vi "MAT_Footer.vi"(6 "byte order":T2(ring)=enum."little-endian", 9 "# plots":i32=6, 10 "frequency":dbl=40000.0, 11 "npts":i32=32768) -> (3 "String":string)   [LabVIEW 2022 SP3]
uses:
  miDataType.ctl
panel:
  out "Array":T1(array[cluster])
  out "WoodhouseCheck":bool
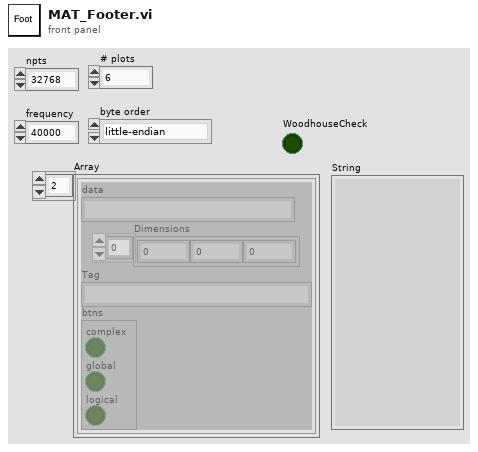
[diagram p1: front panel]
types:
  T1 = cluster{"data":string, "Dimensions":i32[], "Tag":string, "btns":cluster{"complex":bool, "global":bool, "logical":bool}}[]
  T2 = enum16{"big-endian, network order", "native, host order", "little-endian"}
  T3 = cluster{"name":string, "Dimensions":i32[], "Tag":string, "btns":cluster{"complex":bool, "global":bool, "logical":bool}}[]
  T4 = typedef "miDataType.ctl" = enum16{"illegal", "miINT8", "miUINT8", "miINT16", "miUINT16", "miINT32", "miUINT32", "miSINGLE", "--", "miDOUBLE", "---", "----", "miINT64", "miUINT64", "miMATRIX", "miCOMPRESSED", "miUTF8", "miUTF16", "miUTF32", "udefined"}
  T5 = cluster{"data":string, "Dimensions":i32[], "Tag":cluster{"Data Type":T4, "# bytes":u32, "data":string}, "btns":cluster{"complex":bool, "global":bool, "logical":bool}}[]
  T6 = cluster{"Data Type":T4, "# bytes":u32, "data":string}
  T7 = cluster{"name":string, "Dimensions":i32[], "Tag":string, "btns":cluster{"complex":bool, "global":bool, "logical":bool}}
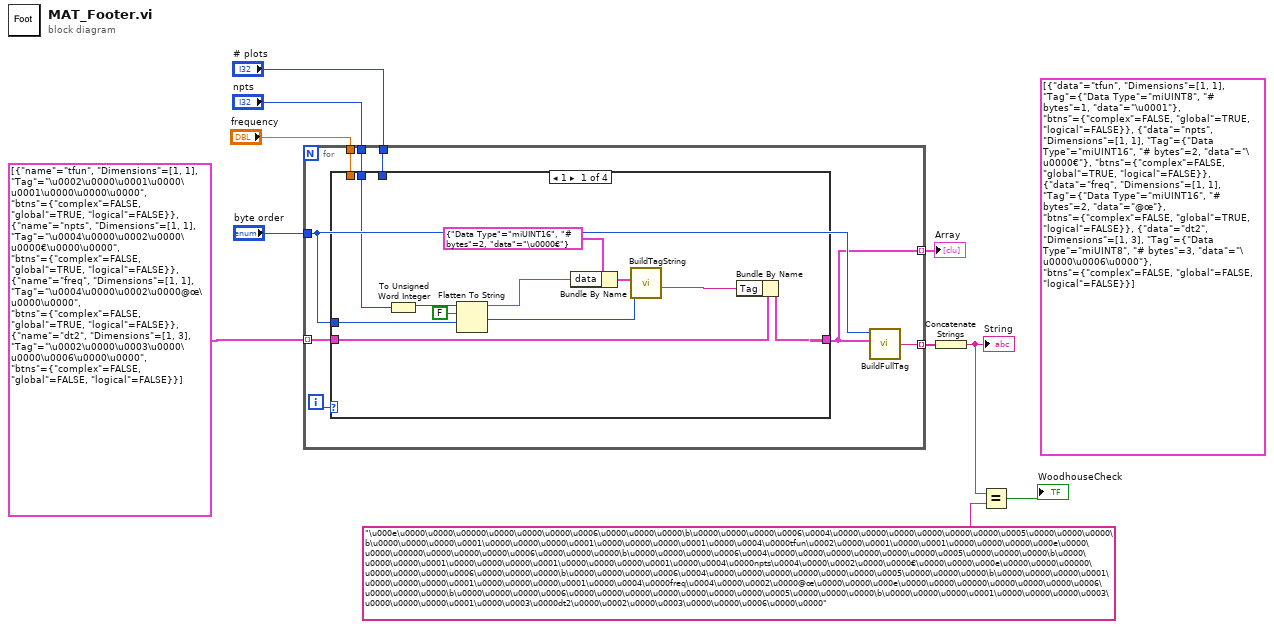
[diagram p0: block diagram]
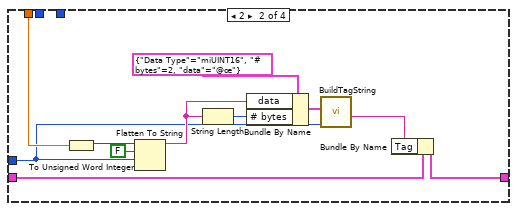
[diagram p2: hidden frame]
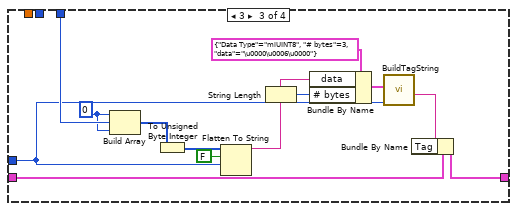
[diagram p3: hidden frame]
diagram:
  (unwired) T5 [{"data"="tfun", "Dimensions"=[1, 1], "Tag"={"Data Type"=enum."miUINT8", "# bytes"=1, "data"="\u0001"}, "btns"={"complex"=FALSE, "global"=TRUE, "logical"=FALSE}}, {"data"="npts", "Dimensions"=[1, 1], "Tag"={"Data Type"=enum."miUINT16", "# bytes"=2, "data"="\u0000€"}, "btns"={"complex"=FALSE, "global"=TRUE, "logical"=FALSE}}, {"data"="freq", "Dimensions"=[1, 1], "Tag"={"Data Type"=enum."miUINT16", "# bytes"=2, "data"="@œ"}, "btns"={"complex"=FALSE, "global"=TRUE, "logical"=FALSE}}, {"data"="dt2", "Dimensions"=[1, 3], "Tag"={"Data Type"=enum."miUINT8", "# bytes"=3, "data"="\u0000\u0006\u0000"}, "btns"={"complex"=FALSE, "global"=FALSE, "logical"=FALSE}}]
  n1 = for {
    tunnel: "byte order" -> [w14]
    tunnel: [w18] -> w6 mode=indexing
    tunnel: T3 [{"name"="tfun", "Dimensions"=[1, 1], "Tag"="\u0002\u0000\u0001\u0000\u0001\u0000\u0000\u0000", "btns"={"complex"=FALSE, "global"=TRUE, "logical"=FALSE}}, {"name"="npts", "Dimensions"=[1, 1], "Tag"="\u0004\u0000\u0002\u0000\u0000€\u0000\u0000", "btns"={"complex"=FALSE, "global"=TRUE, "logical"=FALSE}}, {"name"="freq", "Dimensions"=[1, 1], "Tag"="\u0004\u0000\u0002\u0000@œ\u0000\u0000", "btns"={"complex"=FALSE, "global"=TRUE, "logical"=FALSE}}, {"name"="dt2", "Dimensions"=[1, 3], "Tag"="\u0002\u0000\u0003\u0000\u0000\u0006\u0000\u0000", "btns"={"complex"=FALSE, "global"=FALSE, "logical"=FALSE}}] -> [w16] mode=indexing
    tunnel: "npts" -> [w15]
    tunnel: "frequency" -> [w13]
    tunnel: "# plots" -> [w12]
    tunnel: [w11] -> w2 mode=indexing
    i -> [w17]
    n2 = case shown="1" w17 {
      tunnel: [w27 w38 w51 w53] -> w11
      tunnel: w16 -> [w28 w39 w52 w53]
      tunnel: w15 -> [w26 _ _ _]
      tunnel: w14 -> [w19 w29 w40 _]
      tunnel: w13 -> [_ w35 _ _]
      tunnel: w12 -> [_ _ w48 _]
      frame 1 {
        n3 = To Unsigned Word Integer(number=w26) -> (unsigned 16bit integer=w24:u16)
        n4 = Flatten To String(anything=w24, prepend array or string size? (T)=FALSE ("data includes array or string size? (T)"), byte order (0:big-endian, network order)=w19) -> (data string=w22:string)  [unwired: 1 in, 2 out]
        n5 = Bundle By Name(cluster=T6 {"Data Type"=enum."miUINT16", "# bytes"=2, "data"="\u0000€"} ("Tag"), "data"=w22) -> (w21:T6)
        n6 = call "BuildTagString.vi"("byte order"=w19, "Tag"=w21) -> ("Compressed String Out"=w20:string)  [unwired: 8 in, 1 out]
        n7 = Bundle By Name(cluster=w28, "Tag"=w20) -> (w27:T7)
      }
      frame 2 {
        n8 = To Unsigned Word Integer(number=w35) -> (unsigned 16bit integer=w36:u16)
        n9 = Flatten To String(anything=w36, prepend array or string size? (T)=FALSE ("data includes array or string size? (T)"), byte order (0:big-endian, network order)=w29) -> (data string=w31:string)  [unwired: 1 in, 2 out]
        n10 = String Length(string=w31) -> (length=w34:i32)
        n11 = Bundle By Name(cluster=T6 {"Data Type"=enum."miUINT16", "# bytes"=2, "data"="@œ"} ("Tag"), "data"=w31, "# bytes"=w34) -> (w33:T6)
        n12 = call "BuildTagString.vi"("byte order"=w29, "Tag"=w33) -> ("Compressed String Out"=w30:string)  [unwired: 8 in, 1 out]
        n13 = Bundle By Name(cluster=w39, "Tag"=w30) -> (w38:T7)
      }
      frame 3 {
        w46 = 0
        n14 = Build Array(w46, w48, w46) -> (w47:i32[])
        n15 = To Unsigned Byte Integer(number=w47) -> (unsigned 8bit integer=w49:u8[])
        n16 = Flatten To String(anything=w49, prepend array or string size? (T)=FALSE ("data includes array or string size? (T)"), byte order (0:big-endian, network order)=w40) -> (data string=w42:string)  [unwired: 1 in, 2 out]
        n17 = String Length(string=w42) -> (length=w45:i32)
        n18 = Bundle By Name(cluster=T6 {"Data Type"=enum."miUINT8", "# bytes"=3, "data"="\u0000\u0006\u0000"} ("Tag"), "data"=w42, "# bytes"=w45) -> (w44:T6)
        n19 = call "BuildTagString.vi"("byte order"=w40, "Tag"=w44) -> ("Compressed String Out"=w41:string)  [unwired: 8 in, 1 out]
        n20 = Bundle By Name(cluster=w52, "Tag"=w41) -> (w51:T7)
      }
      frame Default {
      }
    }
    n21 = call "BuildFullTag.vi"("Cluster"=w11, "byte order"=w14) -> ("String Out"=w18:string)  [unwired: 9 in]
  }
  "Array" <- w2
  n22 = Concatenate Strings(w6) -> (w3:string)
  "String" <- w3
  n23 = Equal?(x=w3, y="\u000e\u0000\u0000\u00000\u0000\u0000\u0000\u0006\u0000\u0000\u0000\b\u0000\u0000\u0000\u0006\u0004\u0000\u0000\u0000\u0000\u0000\u0000\u0005\u0000\u0000\u0000\b\u0000\u0000\u0000\u0001\u0000\u0000\u0000\u0001\u0000\u0000\u0000\u0001\u0000\u0004\u0000tfun\u0002\u0000\u0001\u0000\u0001\u0000\u0000\u0000\u000e\u0000\u0000\u00000\u0000\u0000\u0000\u0006\u0000\u0000\u0000\b\u0000\u0000\u0000\u0006\u0004\u0000\u0000\u0000\u0000\u0000\u0000\u0005\u0000\u0000\u0000\b\u0000\u0000\u0000\u0001\u0000\u0000\u0000\u0001\u0000\u0000\u0000\u0001\u0000\u0004\u0000npts\u0004\u0000\u0002\u0000\u0000€\u0000\u0000\u000e\u0000\u0000\u00000\u0000\u0000\u0000\u0006\u0000\u0000\u0000\b\u0000\u0000\u0000\u0006\u0004\u0000\u0000\u0000\u0000\u0000\u0000\u0005\u0000\u0000\u0000\b\u0000\u0000\u0000\u0001\u0000\u0000\u0000\u0001\u0000\u0000\u0000\u0001\u0000\u0004\u0000freq\u0004\u0000\u0002\u0000@œ\u0000\u0000\u000e\u0000\u0000\u00000\u0000\u0000\u0000\u0006\u0000\u0000\u0000\b\u0000\u0000\u0000\u0006\u0000\u0000\u0000\u0000\u0000\u0000\u0000\u0005\u0000\u0000\u0000\b\u0000\u0000\u0000\u0001\u0000\u0000\u0000\u0003\u0000\u0000\u0000\u0001\u0000\u0003\u0000dt2\u0000\u0002\u0000\u0003\u0000\u0000\u0006\u0000\u0000" ("Left")) -> (x = y?=→"WoodhouseCheck":bool)
